vi "Initialise.vi"() -> (3 "Control State out":refnum<class "Control State.lvclass">)   [LabVIEW 2015, in "Control State.lvclass"]
uses:
  Control State.lvclass
  Button State.ctl
  Control State.lvclass/Control State.ctl
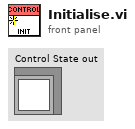
[diagram p1: front panel]
types:
  T1 = typedef "Control State.lvclass/Button State.ctl" = enum16{"Undefined", "Pressed", "Released", "Held", "Not Held"}
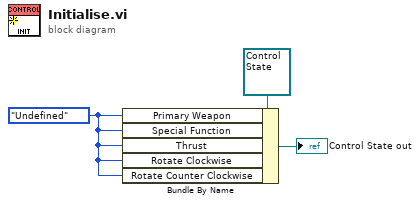
[diagram p0: block diagram]
diagram:
  w1 = Button_State."Undefined" ("Primary Weapon")
  n1 = Bundle By Name(cluster=refnum<class "Control State.lvclass"> refnum ("Control State in"), "Primary Weapon"=w1, "Special Function"=w1, "Thrust"=w1, "Rotate Clockwise"=w1, "Rotate Counter Clockwise"=w1) -> (→"Control State out":refnum<class "Control State.lvclass">)
